vi "test Is Sub-Section_1.vi"(11 "Test Case In":refnum<class "test EDS.lvclass">) -> (0 "error out":errorcluster, 3 "Test Case Out":refnum<class "test EDS.lvclass">)   [LabVIEW 2024, in "test EDS.lvclass"]
uses:
  test EDS.lvclass
  C:/Program Files/National Instruments/LabVIEW 2024/vi.lib/Astemes/LUnit/Test Case.lvclass
  <vilib>/Astemes/LUnit/Test Case.lvclass/Test Case.ctl
  <vilib>/Astemes/LUnit/Append Pass Result.vi
  <vilib>/Astemes/LUnit/Append Fail Result.vi
  <vilib>/Astemes/LUnit/Run In UI.vi
  <vilib>/Utility/error.llb/Clear Errors.vi
  Core/Section Name/Section Name.lvclass
  <vilib>/Astemes/LUnit/Test Case.lvclass
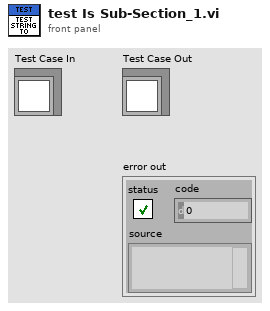
[diagram p1: front panel]
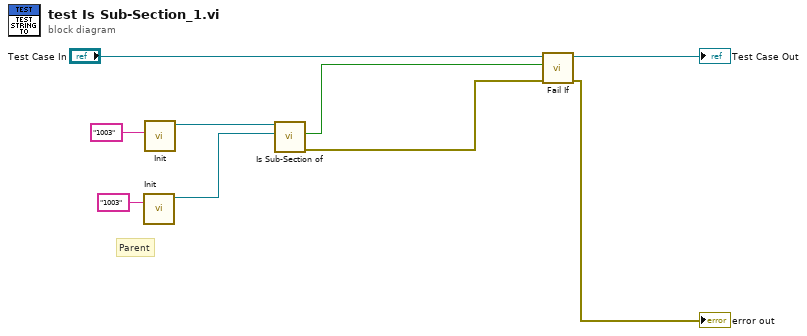
[diagram p0: block diagram]
diagram:
  # "Parent"
  n1 = call "Init.vi"("Section Name"="1003") -> ("Section Name out"=w4:refnum<class "Section Name.lvclass">)  [unwired: 9 in, 1 out]
  n2 = call "Init.vi"("Section Name"="1003") -> ("Section Name out"=w5:refnum<class "Section Name.lvclass">)  [unwired: 9 in, 1 out]
  n3 = call "Is Sub-Section of.vi"("Parent Section Name"=w4, "Section Name in"=w5) -> ("error out"=w6:errorcluster, "Is Sub-Section of?"=w3:bool)  [unwired: 7 in, 1 out]
  n4 = call <vilib>:"Fail If.vi"("error in (no error)"=w6, "Fail?"=w3, "LUnit Test Case In"="Test Case In") -> ("error out"=→"error out":errorcluster, "LUnit Test Case Out"=→"Test Case Out":refnum<class "test EDS.lvclass">)  [unwired: 7 in]
